vi "MainRT.vi"() -> ()   [LabVIEW 2017]
doc: "The myRIO Project template acquires acceleration data from the onboard accelerometer and displays the changes of acceleration values in a waveform chart."
uses:
  Controls/DataStreamCluster.ctl
  Controls/CommandsRT.ctl
  <vilib>/myRIO/Instrument Drivers/Onboard IO/DIO/typedefs/DIO Reference.ctl
  <vilib>/myRIO/Common/Instrument Driver Framework/Utilities/typedefs/myRIO Generic Hardware Reference.ctl
  <vilib>/myRIO/Common/Instrument Driver Framework/Utilities/typedefs/Hardware Version Enum.ctl
  <vilib>/myRIO/Common/Instrument Driver Framework/Utilities/typedefs/myRIO v1.0 Reference.ctl
  <vilib>/myRIO/Common/Instrument Driver Framework/Utilities/typedefs/Generic FPGA Reference.ctl
  <vilib>/myRIO/Common/Instrument Driver Framework/myRIO v1.0/DIO/typedefs/DIO Channels List.ctl
  <vilib>/myRIO/Common/Instrument Driver Framework/myRIO v1.0/DIO/typedefs/DIO Channels Enum.ctl
  <vilib>/userdefined/High Color/nirio_resource_hc.ctl
  <vilib>/myRIO/Common/Instrument Driver Framework/Utilities/vis/Is FPGA Ref Available.vi
  <vilib>/myRIO/Common/Instrument Driver Framework/myRIO v1.0/DIO/vis/myRIO v1.1 Open DIO.vi
  <extravilib>/ChannelInstances/Tag-t'DataStreamCluster.ctl'/Write With Abort.vi
  <vilib>/myRIO/Common/Instrument Driver Framework/myRIO v1.0/UART/vis/myRIO v1.0 Close UART.vi
  <extravilib>/ChannelInstances/Tag-t'DataStreamCluster.ctl'/Read With Abort.vi
  <vilib>/myRIO/Common/Instrument Driver Framework/Utilities/vis/Validate Channels.vi
  <vilib>/myRIO/Common/Instrument Driver Framework/myRIO v1.0/DIO/vis/myRIO v1.0 Reserve DIO.vi
  <vilib>/myRIO/Common/Instrument Driver Framework/myRIO v1.0/Resource Manager/vis/myRIO v1.0 Reserve Channel List.vi
  <vilib>/myRIO/Common/Instrument Driver Framework/myRIO v1.0/DIO/vis/myRIO v1.0 Build MUX Configuration DIO.vi
  <vilib>/myRIO/Common/Instrument Driver Framework/myRIO v1.0/Resource Manager/vis/myRIO v1.0 Reserve Channel.vi
  <vilib>/myRIO/Common/Instrument Driver Framework/myRIO v1.0/Resource Manager/vis/myRIO v1.0 Unreserve Channel.vi
  <vilib>/myRIO/Common/Instrument Driver Framework/myRIO v1.0/Resource Manager/vis/myRIO v1.0 Create Configuration List.vi
  <vilib>/myRIO/Common/Instrument Driver Framework/myRIO v1.0/Resource Manager/vis/myRIO v1.0 Build Mutex Name.vi
  <extravilib>/ChannelInstances/Tag-t'DataStreamCluster.ctl'/Instantiate.vi
  <extravilib>/ChannelInstances/Tag-t'DataStreamCluster.ctl'/EndpointRead.vi
  <vilib>/Utility/VariantDataType/GetNumericInfo.vi
  <vilib>/Utility/error.llb/Error Cluster From Error Code.vi
  <vilib>/myRIO/Common/Instrument Driver Framework/myRIO v1.0/myRIO v1.1 Open.vi
  <vilib>/myRIO/Common/Instrument Driver Framework/Utilities/vis/IO Manager.vi
  <vilib>/myRIO/Common/Instrument Driver Framework/Utilities/vis/Configuration Manager.vi
  <vilib>/myRIO/Common/Instrument Driver Framework/myRIO v1.0/Resource Manager/vis/myRIO v1.0 Configure IO.vi
  <vilib>/myRIO/Common/Instrument Driver Framework/myRIO v1.0/myRIO v1.0 Close.vi
  <vilib>/myRIO/Common/Instrument Driver Framework/myRIO v1.0/DIO/vis/myRIO v1.0 Write DIO.vi
  <extravilib>/ChannelInstances/Tag-t'DataStreamCluster.ctl'/Endpoint.vi
  <vilib>/myRIO/Common/Instrument Driver Framework/Utilities/vis/FPGA Ref Manager.vi
  <vilib>/myRIO/Common/Instrument Driver Framework/myRIO v1.0/myRIO v1.0 Reset FPGA.vi
  <vilib>/myRIO/Common/Instrument Driver Framework/myRIO v1.0/IRQ/vis/myRIO v1.0 IRQ Info FGV.vi
  <vilib>/myRIO/Common/Instrument Driver Framework/myRIO v1.0/IRQ/vis/myRIO v1.0 Timer IRQ Info FGV.vi
  <vilib>/myRIO/Common/Instrument Driver Framework/myRIO v1.0/IRQ/vis/myRIO v1.0 ISR Agent.vi
  <vilib>/myRIO/Express VI/Onboard Devices/LED/LED Express VI.xnode
  <vilib>/myRIO/Instrument Drivers/Onboard IO/DIO/vis/myRIO DIO Open.xnode
  <vilib>/myRIO/Instrument Drivers/Utilities/Utilities.lvlib
  <vilib>/myRIO/Instrument Drivers/Onboard IO/DIO/DIO.lvlib
  <extravilib>/ChannelInstances/Tag-t'DataStreamCluster.ctl'.lvlib
panel:
  out "Stop":bool
  out "Pause":bool
  out "Start":bool
  out "element":T1
  out "data out":T2
  out "error out":errorcluster
  # "Overview\nMainRT receives commands fro PC via Network Streams.\n\nInstructions"
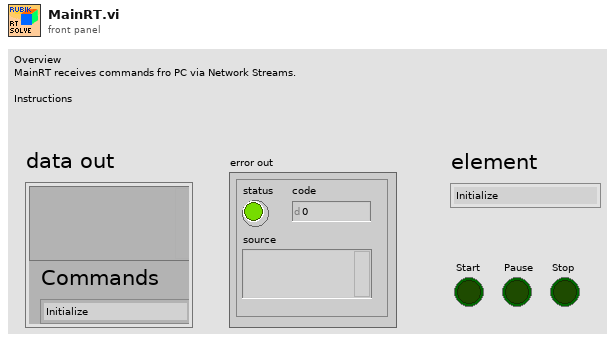
[diagram p1: front panel]
types:
  T1 = typedef "CommandsRT.ctl" = enum16{"Initialize", "Start", "Pause", "Stop", "Exit"}
  T2 = typedef "DataStreamCluster.ctl" = cluster{"Commands":T1, variant}
  T3 = typedef "Tag-t'DataStreamCluster.ctl'.lvlib/))Channel.ctl" = refnum<queue>
  T4 = typedef "DIO.lvlib/DIO Reference.ctl" = cluster{"myRIO Reference":T5, "DIO Channels List":T9}
  T5 = typedef "myRIO Generic Hardware Reference.ctl" = cluster{"myRIO Model":T6, "myRIO Hardware Reference":T7}
  T6 = typedef "Hardware Version Enum.ctl" = enum16{"Unknown", "myRIO-1900", "myRIO-1950", "roboRIO", "NI ELVIS RIO CM"}
  T7 = typedef "myRIO v1.0 Reference.ctl" = cluster{"Generic FPGA Reference":T8, "Allow multiple opens":bool}
  T8 = typedef "Generic FPGA Reference.ctl" = refnum<k20>
  T9 = typedef "DIO Channels List.ctl" = T10[]
  T10 = typedef "DIO Channels Enum.ctl" = enum16{"Not Connected", "C/DIO0", "C/DIO1", "C/DIO2", "C/DIO3", "C/DIO4", "C/DIO5", "C/DIO6", "C/DIO7", "A/DIO0", "A/DIO1", "A/DIO2", "A/DIO3", "A/DIO4", "A/DIO5", "A/DIO6", "A/DIO7", "A/DIO8", "A/DIO9", "A/DIO10", "A/DIO11", "A/DIO12", "A/DIO13", "A/DIO14", "A/DIO15", "B/DIO0", "B/DIO1", "B/DIO2", "B/DIO3", "B/DIO4", "B/DIO5", "B/DIO6", "B/DIO7", "B/DIO8", "B/DIO9", "B/DIO10", "B/DIO11", "B/DIO12", "B/DIO13", "B/DIO14", "B/DIO15", "LED0", "LED1", "LED2", "LED3", "Button0", "DIO/DIO0", "DIO/DIO1", "DIO/DIO2", "DIO/DIO3", "DIO/DIO4", "DIO/DIO5", "DIO/DIO6", "DIO/DIO7", "DIO/DIO8", "DIO/DIO9", "SPI/CS0", "SPI/CS1", "SPI/CS2", "SPI/CS3", "LED RADIO (Green)", "LED RADIO (Red)", "LED COMM (Green)", "LED COMM (Red)", "LED MODE (Green)", "LED MODE (Red)"}
  T11 = typedef "nirio_resource_hc.ctl" = tag
  T12 = typedef "OrientationState.ctl" = enum16{"FrontState", "UpState", "BackState", "DownState"}
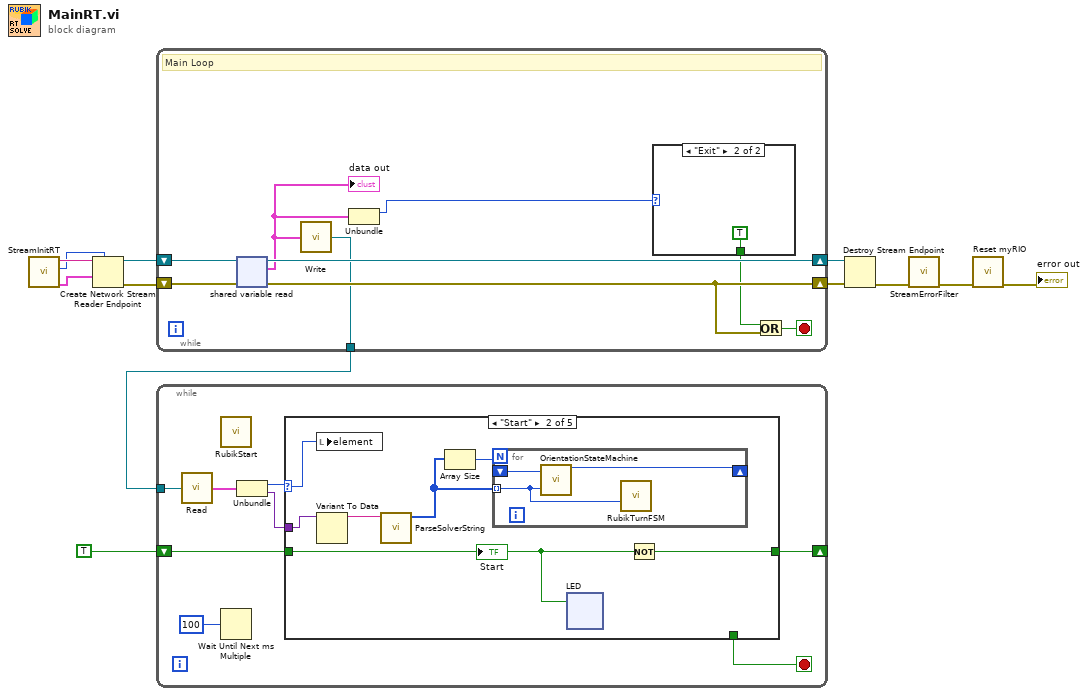
[diagram p0: block diagram]
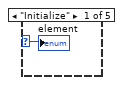
[diagram p2: hidden frame]
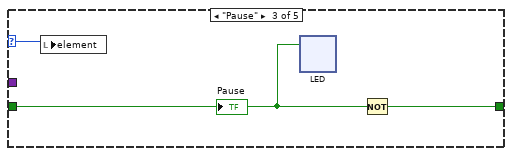
[diagram p3: hidden frame]
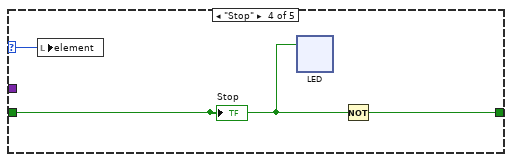
[diagram p4: hidden frame]
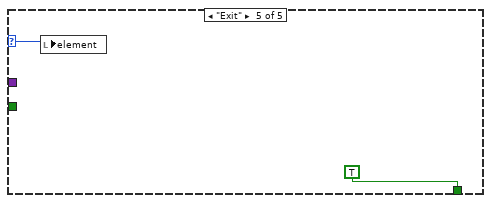
[diagram p5: hidden frame]
diagram:
  n1 = call "StreamInitRT.vi"() -> ("data type"=w5:T2, "reader buffer size"=w11:i32, "reader name"=w12:string)  [unwired: 9 in]
  n2 = Create Network Stream Reader Endpoint(7:w11, 9:w5, 11:w12) -> (0:w10:errorcluster, 3:w9:refnum<k21>)  [unwired: 4 in]
  n3 = while {
    shift-right: [w19] -> w6
    shift-left: w10 -> [w19]
    shift-right: [w17] -> w7
    shift-left: w9 -> [w18]
    tunnel: [w13] -> w1
    stop <- w20 stop-if-true
    # "Main Loop"
    n4 = shared-variable-read(w18) -> (w17:refnum<k21>, w14:T2)  [unwired: 2 in, 2 out]
    "data out" <- w14
    n5 = call <vilib>:"Write.vi"("element"=w14) -> ("channel"=w13:T3)  [unwired: 1 out]
    n6 = Unbundle(w14) -> ("Commands"=w16:T1)  [unwired: 1 out]
    n7 = case shown="\"Exit\"" w16 {
      tunnel: [_ TRUE] -> w15
      frame "Initialize".."Stop" {
      }
      frame "Exit" {
      }
    }
    n8 = Or(x=w15, y=w19) -> (x .or. y?=w20:bool)
  }
  n9 = while {
    shift-right: [w27] -> _
    shift-left: TRUE -> [w28]
    tunnel: w1 -> [w25]
    stop <- w29 stop-if-true
    n10 = call <extravilib>:"Read.vi"("channel"=w25) -> ("element"=w24:T2)  [unwired: 1 in, 1 out]
    n11 = call "RubikStart.vi"() -> ()  [unwired: 12 in]
    n12 = Wait Until Next ms Multiple(millisecond multiple=u32 100) -> ()  [unwired: 1 out]
    n13 = Unbundle(w24) -> ("Commands"=w23:T1, w22:variant)
    n14 = case shown="\"Start\"" w23 {
      selector: w23 -> [w30 w37 w78 w116 w152]
      tunnel: [_ _ _ _ TRUE] -> w29
      tunnel: w28 -> [_ w35 w76 w114 _]
      tunnel: [_ w36 w77 w115 _] -> w27
      tunnel: w22 -> [_ w34 _ _ _]
      frame "Initialize" {
        "element" <- w30
      }
      frame "Start" {
        n15 = local write "element"(w37) -> ()
        n16 = Variant To Data(Variant=w34) -> (data=w33:string)  [unwired: 2 in, 1 out]
        n17 = call "ParseSolverString.vi"("String"=w33) -> ("Array"=w31:u16[])  [unwired: 10 in]
        n18 = Array Size(array=w31) -> (size(s)=w32:i32)
        n19 = for {
          N: w32 -> [_]
          tunnel: w31 -> [w38] mode=indexing
          shift-right: [w39] -> _
          shift-left: _ -> [w40]
          n20 = call "OrientationStateMachine.vi"("Rubik's Moves"=w38, "Initial Orientation"=w40) -> ("Final Orientation"=w39:T12)  [unwired: 9 in]
          n21 = call "RubikTurnFSM.vi"("Turn"=w38) -> ()  [unwired: 1 in]
        }
        n22 = xnode "LED"("LED0"=w35) -> ()  [unwired: 1 in, 1 out]
        n23 = Not(x=w35) -> (.not. x?=w36:bool)
        "Start" <- w35
      }
      frame "Pause" {
        n24 = local write "element"(w78) -> ()
        n25 = xnode "LED"("LED1"=w76) -> ()  [unwired: 1 in, 1 out]
        n26 = Not(x=w76) -> (.not. x?=w77:bool)
        "Pause" <- w76
      }
      frame "Stop" {
        n27 = local write "element"(w116) -> ()
        n28 = xnode "LED"("LED2"=w114) -> ()  [unwired: 1 in, 1 out]
        n29 = Not(x=w114) -> (.not. x?=w115:bool)
        "Stop" <- w114
      }
      frame "Exit" {
        n30 = local write "element"(w152) -> ()
      }
    }
  }
  n31 = Destroy Stream Endpoint(8:w6, 11:w7) -> (0:w8:errorcluster)
  n32 = call "StreamErrorFilter.vi"("error in (no error)"=w8) -> ("error out"=w3:errorcluster)  [unwired: 10 in]
  n33 = call <vilib>:"Reset myRIO.vi"("error in (no error)"=w3) -> ("error out"=→"error out":errorcluster)  [unwired: 10 in]
